vi "Read Command.vi"(8 "error in (no error)":errorcluster, 11 "Connection ID in":refnum<k5>) -> (0 "error out":errorcluster, 3 "Connection ID out":refnum<k5>)   [LabVIEW 2015]
uses:
  Relay State.ctl
  <vilib>/Espotel/IoT Foundation/IoTF/IoTF Library.lvlib
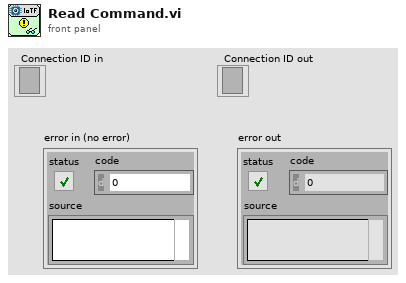
[diagram p1: front panel]
types:
  T1 = typedef "Relay State.ctl" = cluster{"Relay State":bool}
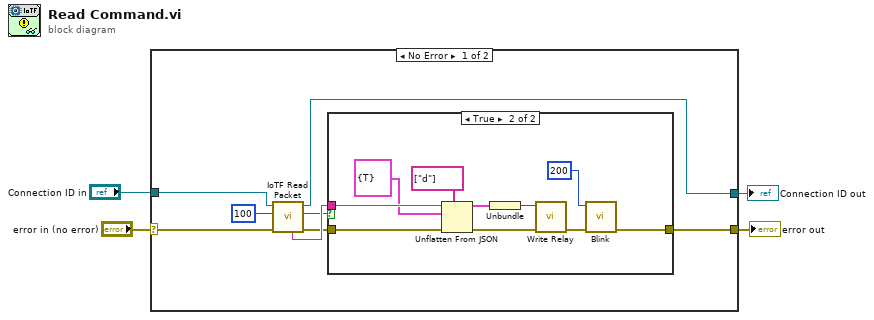
[diagram p0: block diagram]
diagram:
  n1 = case shown="No Error" "error in (no error)" {
    selector: "error in (no error)" -> [w6 w25]
    tunnel: [w8 w24] -> w1
    tunnel: [w7 w25] -> w4
    tunnel: "Connection ID in" -> [w5 w24]
    frame No Error {
      n2 = call <vilib>:"IoTF Read Packet.vi"("Error in (no error)"=w6, "Timeout (10000ms)"=100, "Connection ID in"=w5) -> ("Error out"=w11:errorcluster, "Packet Arrived?"=w10:bool, "Connection ID out"=w8:refnum<k5>, "Message"=w12:string)  [unwired: 4 in, 1 out]
      n3 = case shown="True" w10 {
        tunnel: w12 -> [_ w21]
        tunnel: w11 -> [w13 w16]
        tunnel: [w13 w15] -> w7
        frame False {
        }
        frame True {
          n4 = Unflatten From JSON(path=string[] ["d"], JSON string=w21, type and defaults=T1 {"Relay State"=TRUE} ("d"), error in (no error)=w16) -> (value=w19:T1, error out=w17:errorcluster)  [unwired: 3 in]
          n5 = Unbundle(w19) -> ("Relay State"=w18:bool)
          n6 = call "Write Relay.vi"("error in (no error)"=w17, "status"=w18) -> ("error out"=w23:errorcluster)  [unwired: 9 in]
          n7 = call "Blink.vi"("error in (no error)"=w23, "milliseconds to wait (100)"=u32 200) -> ("error out"=w15:errorcluster)  [unwired: 9 in]
        }
      }
    }
    frame Error {
    }
  }
  "error out" <- w4
  "Connection ID out" <- w1
